vi "AngleMultiplier_Wrapping.vi"(10 "Multiplier (M)":fxp<+/-,18,6>, 11 "Input angle (x)":fxp<+/-,25,1>) -> (3 "Output angle (y)":fxp<+/-,25,1> format="%#.6g")   [LabVIEW 2020, in "FPGA functions.lvlib"]
doc: "Multiplies input angle (x) by multiplier (M) and wraps the output angle (y = Mx) within the range -1 to 1 (pi radians).\n\nInput is in pi radians (domain of x is -1 to 1), that is angle is from -pi to pi. \n\nOutput is in pi radians (range of y is -1 to 1), that is angle is from -pi to pi."
uses:
  FPGA functions.lvlib
  <vilib>/Platform/TimedLoop/XDataNode/timing_clust.ctl
  <vilib>/Platform/TimedLoop/XDataNode/nitl_modes.ctl
  <vilib>/Platform/TimedLoop/XDataNode/wakeup.ctl
  <vilib>/rvi/Emulation/niFpgaSctlEmulationGetInTimedLoop.vi
  <vilib>/rvi/Emulation/niFpgaEmulationReportErrorSimple.vi
  <vilib>/rvi/Emulation/niFpgaGetClockAttributes.vi
  <vilib>/rvi/Emulation/niFpgaCriticalErrorInLSC.vi
  <vilib>/Platform/TimedLoop/XDataNode/XDataNode.xnode
  <vilib>/rvi/FXPMathLib/FxpMul/XNode/nifxpmath_Multiplier.xnode
  <vilib>/rvi/FXPMathLib/FxpSub/XNode/nifxpmath_Sub.xnode
  <vilib>/Platform/TimedLoop/XDataNode/XDNodeRunTimeDep.lvlib
  <vilib>/rvi/FXPMathLib/sim/FxpSim.dll
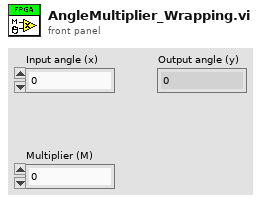
[diagram p1: front panel]
types:
  T1 = typedef "XDNodeRunTimeDep.lvlib/timing_clust.ctl" = cluster{"Expected End [f-1]":u64, "Actual End [f-1]":u64, "Finished Late? [f-1]":bool, "Expected End [i-1]":u64, "Actual End [i-1]":u64, "Finished Late? [i-1]":bool, "Expected Start [i]":u64, "Actual Start [i]":u64, "Expected Start [f]":u64, "Actual Start [f]":u64, "Source Name":string, "Structure Name":string, "Period":i64, "Deadline":i64, "Offset":i64, "Start":i64, "Priority":i32, "Timeout":i32, "Mode":T2, "Wakeup Reason":T3, "Error":errorcluster, "Source Type":string, "Secondary Source Type":string, "Global End Time":u64, "Global Start Time":u64, "Frame Duration":u64, "Iteration Duration":u64, "Assigned CPU":i32, "I/O Scan Engine Mode":u32}
  T2 = typedef "XDNodeRunTimeDep.lvlib/nitl_modes.ctl" = enum32{"No Change", "Process missed periods, maintain original phase", "Discard missed periods, maintain original phase", "Process missed periods, ignore original phase", "Discard missed periods, ignore original phase"}
  T3 = typedef "XDNodeRunTimeDep.lvlib/wakeup.ctl" = enum32{"Normal", "Aborted", "Asynchronous wakeup", "Timing source error", "Timed loop error", "Timeout"}
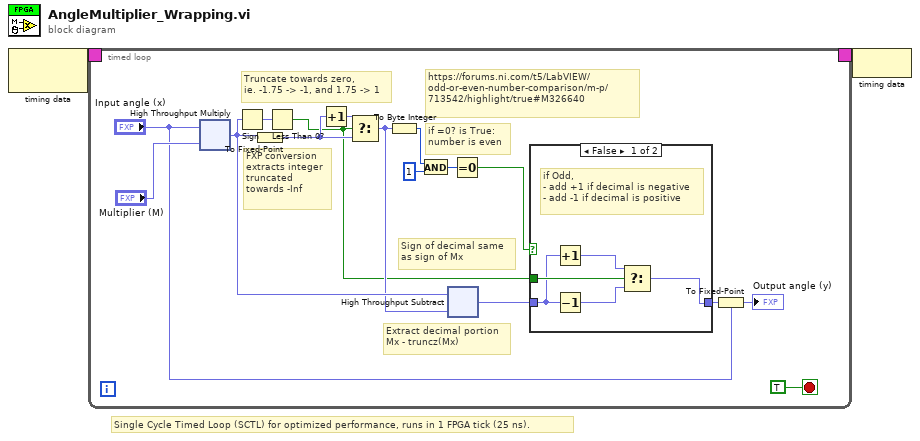
[diagram p0: block diagram]
diagram:
  # "Single Cycle Timed Loop (SCTL) for optimized performance, runs in 1 FPGA tick (25 ns)."
  n1 = node-c288() -> (w2:T1)  [unwired: 1 in]
  n2 = timed-loop {
    timing: w2 -> [_]
    timing-out: [_] -> w1
    stop <- TRUE stop-if-true
    # "FXP conversion\nextracts integer \ntruncated\ntowards -Inf"
    # "https://forums.ni.com/t5/LabVIEW/odd-or-even-number-comparison/m-p/713542/highlight/true#M326640"
    # "Sign of decimal same\nas sign of Mx"
    # "Extract decimal portion\nMx - truncz(Mx)"
    # "Truncate towards zero, \nie. -1.75 -> -1, and 1.75 -> 1"
    # "if =0? is True:\nnumber is even"
    n3 = xnode ("High Throughput Multiply")("x"="Input angle (x)", "y"="Multiplier (M)") -> ("x*y"=w11:fxp<+/-,32,7>)
    n4 = Sign(1:w11) -> (0:w14:fxp<+/-,2,2>)
    n5 = To Fixed-Point(number=w11) -> (fixed-point=w9:fxp<+/-,6,6>)  [unwired: 1 in]
    n6 = Less Than 0?(x=w14) -> (x < 0?=w3:bool)
    n7 = Increment(x=w9) -> (x+1=w13:fxp<+/-,7,7>)
    n8 = Select(t=w13, s=w3, f=w9) -> (s? t:f=w10:fxp<+/-,7,7>)
    n9 = To Byte Integer(number=w10) -> (8bit integer=w8:i8)
    n10 = And(x=w8, y=i8 1) -> (x .and. y?=w15:i8)
    n11 = xnode "High Throughput Subtract"("x"=w11, "y"=w10) -> ("x-y"=w7:fxp<+/-,26,1>)
    n12 = Equal To 0?(x=w15) -> (x = 0?=w12:bool)
    n13 = case shown="False" w12 {
      tunnel: w7 -> [w22 w24]
      tunnel: [w19 w24] -> w6
      tunnel: w3 -> [w23 _]
      frame False {
        # "if Odd,\n- add +1 if decimal is negative\n- add -1 if decimal is positive"
        n14 = Increment(x=w22) -> (x+1=w21:fxp<+,26,1>)
        n15 = Decrement(x=w22) -> (x-1=w20:fxp<+/-,27,2>)
        n16 = Select(t=w21, s=w23, f=w20) -> (s? t:f=w19:fxp<+/-,27,2>)
      }
      frame True {
        # "If Even, pass the decimal \nportion with the sign as is"
      }
    }
    n17 = To Fixed-Point(fixed-point type="Input angle (x)", number=w6) -> (fixed-point=→"Output angle (y)":fxp<+/-,25,1>)
  }
  n18 = node-c288(w1) -> ()
